vi "Create SNS Topic and Email Subscription.vi"() -> ()   [LabVIEW 2015]
doc: "Demonstrates how to create an SNS topic, and then subscribe to that topic with a specified email address."
uses:
  <vilib>/AWS Toolkit/Core/HTTP Request/Region.ctl
  <vilib>/AWS Toolkit/Core/HTTP Request/AWS Credentials.ctl
  <vilib>/AWS Toolkit/SNS/Subscription/Subscription Protocol.ctl
  <vilib>/AWS Toolkit/Core/HTTP Request/HTTP Request.lvclass
  <vilib>/AWS Toolkit/SNS/Topic/Topic.lvclass
  <vilib>/AWS Toolkit/SNS/Subscription/Subscription.lvclass
panel:
  in  "Email Address":string
  in  "Region":T1
  in  "Secret Key":string
  in  "Access Key":string
  in  "Topic Name":string
  # "Overview: Demonstrates how to create an SNS topic, and then subscribe to that topic with a specified email address.\nRequirements: NI Cloud Toolkit for AWS and a registered Amazon AWS account\nInstructions:\n1. Specify the Access Key and Secret Key for your AWS account. You can create an account at http://aws.amazon.com.\n2. Specify a Topic Name for the new SNS topic.\n3. Specify an Email Address to be subscribed to the new SNS topic.\n4. Run the VI. You should receive a confirmation email at the specified email address within a few minutes after running the VI."
  # "Note: Topic names must be globally unique."
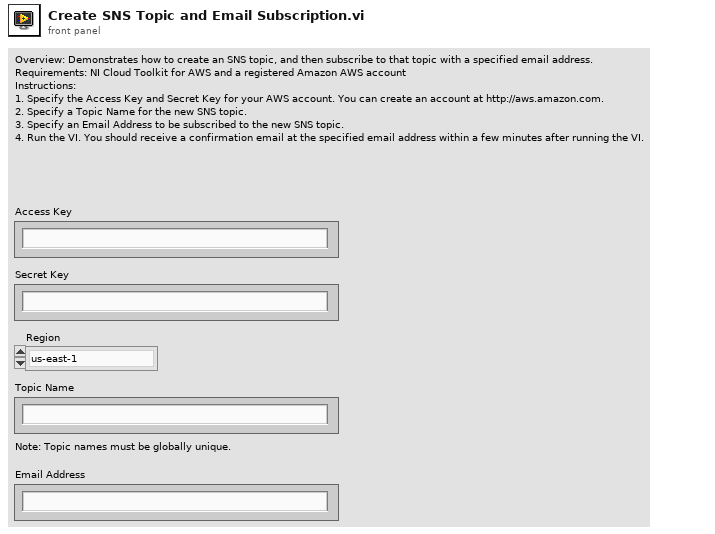
[diagram p1: front panel]
types:
  T1 = typedef "NI_AWS_Core.lvlib/HTTP Request.lvclass/Region.ctl" = enum16{"us-east-1", "us-east-2", "us-west-1", "us-west-2", "ap-northeast-1", "ap-northeast-2", "ap-southeast-1", "ap-southeast-2", "ca-central-1", "eu-central-1", "eu-west-1", "eu-west-2", "sa-east-1"}
  T2 = typedef "NI_AWS_SNS.lvlib/Subscription.lvclass/Subscription Protocol.ctl" = enum16{"http", "https", "email", "email-json", "sms", "sqs", "application", "lambda"}
  T3 = typedef "NI_AWS_Core.lvlib/HTTP Request.lvclass/AWS Credentials.ctl" = cluster{"Access Key":string, "Secret Key":string}
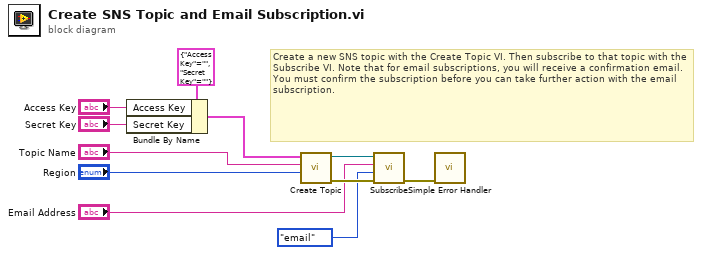
[diagram p0: block diagram]
diagram:
  # "Create a new SNS topic with the Create Topic VI. Then subscribe to that topic with the Subscribe VI. Note that for email subscriptions, you will receive a confirmation email. You must confirm the subscription before you can take further action with the email subscription."
  n1 = Bundle By Name(cluster=T3 {"Access Key"="", "Secret Key"=""} ("AWS Credentials"), "Access Key"="Access Key", "Secret Key"="Secret Key") -> (w8:T3)
  n2 = call <vilib>:"Create Topic.vi"("Region"="Region", "Name"="Topic Name", "AWS Credentials"=w8) -> ("error out"=w5:errorcluster, "Topic out"=w2:refnum<class "Topic.lvclass">)  [unwired: 7 in]
  n3 = call <vilib>:"Subscribe.vi"("error in (no error)"=w5, "Protocol"=Subscription_Protocol."email", "Endpoint"="Email Address", "Topic in"=w2) -> ("error out"=w4:errorcluster)  [unwired: 5 in, 2 out]
  n4 = call <vilib>:"Simple Error Handler.vi"("error in (no error)"=w4) -> ()  [unwired: 4 in, 5 out]
